vi "Read Block.vi"(8 "error in (no error)":errorcluster, 11 "Scope5761":refnum<class "Scope5782_six_channel.lvclass">) -> (0 "error out":errorcluster, 1 "#elements":i32, 2 "Data":dbl[][](array[numeric]), 3 "Scope5761":refnum<class "Scope5782_six_channel.lvclass">, 4 "FFT buffer":dbl[][](array[numeric]))   [LabVIEW 2025, in "Scope5782_six_channel.lvclass"]
uses:
  Scope5782_six_channel.lvclass
  controls/host_transfer_speed.ctl
  ScopeBase/ScopeBase.lvclass/ScopeBase.ctl
  Scope5782_six_channel.lvclass/Scope5782_six_channel.ctl
  FpgaRef/FpgaRef5761/FpgaRef5761.lvclass
  FpgaRef/FpgaRef5782/FpgaRef5782.lvclass
  ScopeBase/ScopeBase.lvclass
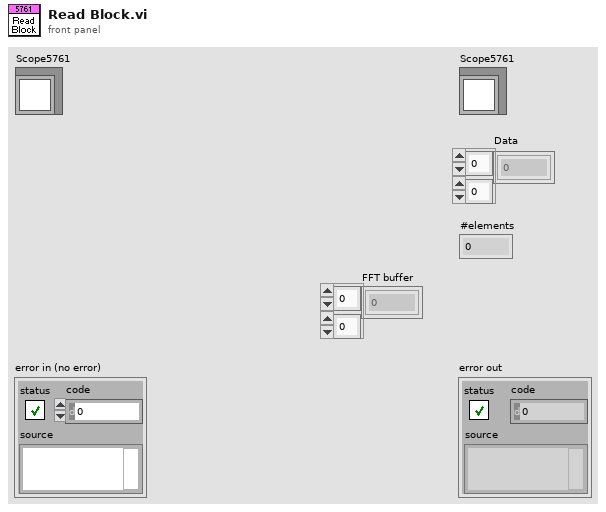
[diagram p1: front panel]
types:
  T1 = typedef "host_transfer_speed.ctl" = enum16{"Very high speed (10Ms/s)", "High speed (1Ms/s)", "Low speed (50kS/s)", "Ultra low speed (20kS/s)"}
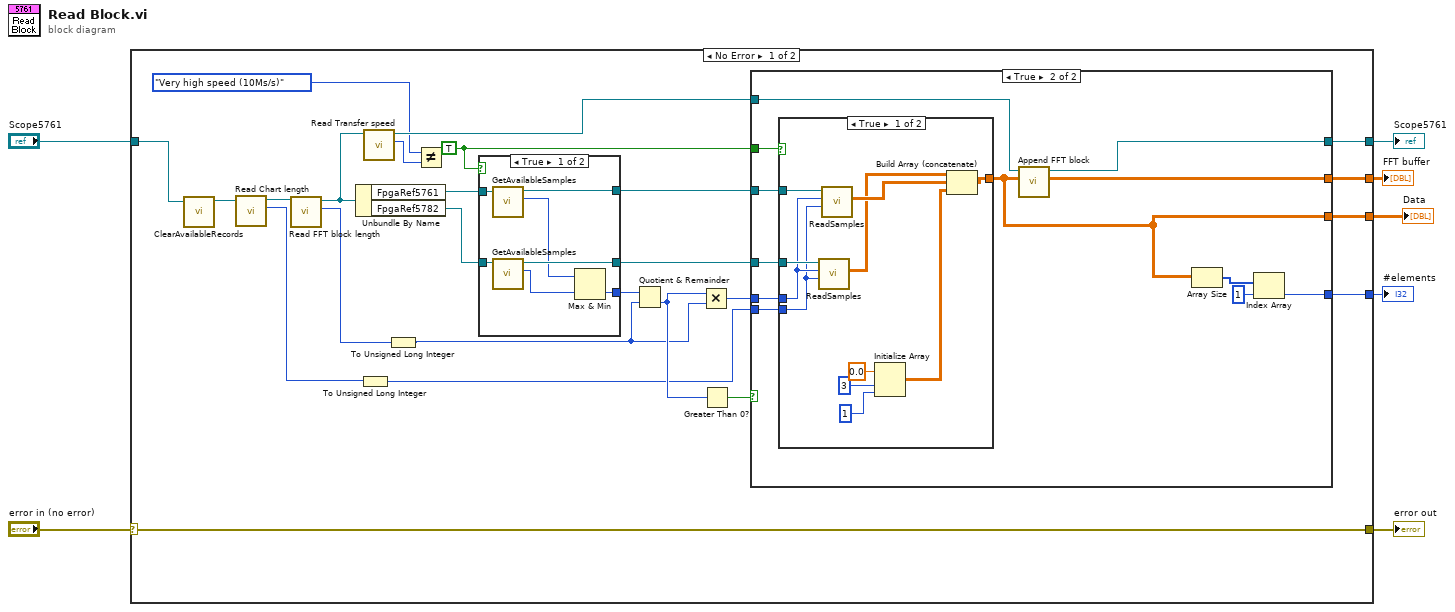
[diagram p0: block diagram]
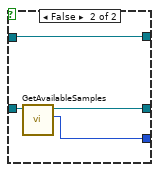
[diagram p2: hidden frame]
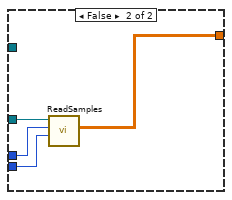
[diagram p4: hidden frame]
diagram:
  n1 = case shown="No Error" "error in (no error)" {
    selector: "error in (no error)" -> [w32 w73]
    tunnel: [w32 w73] -> w6
    tunnel: [w16 w72] -> w4
    tunnel: "Scope5761" -> [w25 w72]
    tunnel: [w31 _] -> w3
    tunnel: [w30 _] -> w2
    tunnel: [w15 _] -> w1
    frame No Error {
      w8 = TRUE
      n2 = call "ClearAvailableRecords.vi"("Scope5785_six_channel"=w25) -> ("Scope5785_six_channel out"=w23:refnum<class "Scope5782_six_channel.lvclass">)  [unwired: 9 in, 1 out]
      n3 = call "Read Chart length.vi"("ScopeBase in"=w23) -> ("Chart length"=w18:i32, "ScopeBase out"=w22:refnum<class "Scope5782_six_channel.lvclass">)  [unwired: 8 in, 1 out]
      n4 = call "Read FFT block length.vi"("ScopeBase in"=w22) -> ("FFT block length"=w14:i32, "ScopeBase out"=w12:refnum<class "Scope5782_six_channel.lvclass">)  [unwired: 8 in, 1 out]
      n5 = Unbundle By Name(w12) -> ("FpgaRef5761"=w29:refnum<class "FpgaRef5761.lvclass">, "FpgaRef5782"=w28:refnum<class "FpgaRef5782.lvclass">)
      n6 = To Unsigned Long Integer(number=w18) -> (unsigned 32bit integer=w17:u32)
      n7 = call "Read Transfer speed.vi"("ScopeBase in"=w12) -> ("Tranfer speed"=w10:T1, "ScopeBase out"=w11:refnum<class "Scope5782_six_channel.lvclass">)  [unwired: 8 in, 1 out]
      n8 = To Unsigned Long Integer(number=w14) -> (unsigned 32bit integer=w13:u32)
      n9 = Not Equal?(x=host_transfer_speed."Very high speed (10Ms/s)" ("y"), y=w10) -> ()  [unwired: 1 out]
      n10 = case shown="True" w8 {
        tunnel: w29 -> [w39 w41]
        tunnel: w28 -> [w38 w43]
        tunnel: [w36 w41] -> w27
        tunnel: [w35 w42] -> w26
        tunnel: [w33 w40] -> w24
        frame True {
          n11 = call-dynamic "GetAvailableSamples.vi"("FpgaRef5761 In"=w39) -> ("available"=w34:u32, "FpgaRef5761 Out"=w36:refnum<class "FpgaRef5761.lvclass">)  [unwired: 8 in, 1 out]
          n12 = call-dynamic "GetAvailableSamples.vi"("FpgaRef5782 in"=w38) -> ("available"=w37:u32, "FpgaRef5782 out"=w35:refnum<class "FpgaRef5782.lvclass">)  [unwired: 8 in, 1 out]
          n13 = Max & Min(x=w34, y=w37) -> (min(x,y)=w33:u32)  [unwired: 1 out]
        }
        frame False {
          n14 = call-dynamic "GetAvailableSamples.vi"("FpgaRef5782 in"=w43) -> ("available"=w40:u32, "FpgaRef5782 out"=w42:refnum<class "FpgaRef5782.lvclass">)  [unwired: 8 in, 1 out]
        }
      }
      n15 = Quotient & Remainder(x=w24, y=w13) -> (floor(x/y)=w20:u32)  [unwired: 1 out]
      n16 = Multiply(x=w20, y=w13) -> (x*y=w19:u32)
      n17 = Greater Than 0?(x=w20) -> (x > 0?=w21:bool)
      n18 = case shown="True" w21 {
        tunnel: [_ w47] -> w31
        tunnel: [_ w54] -> w30
        tunnel: w19 -> [_ w51]
        tunnel: w17 -> [_ w50]
        tunnel: w27 -> [_ w53]
        tunnel: w26 -> [_ w52]
        tunnel: w11 -> [w44 w49]
        tunnel: [w44 w48] -> w16
        tunnel: [_ w46] -> w15
        tunnel: w8 -> [_ w45]
        frame False {
        }
        frame True {
          n19 = case shown="True" w45 {
            tunnel: w53 -> [w67 _]
            tunnel: w52 -> [w66 w71]
            tunnel: w51 -> [w65 w70]
            tunnel: w50 -> [w62 w69]
            tunnel: [w61 w68] -> w47
            frame True {
              n20 = call-dynamic "ReadSamples.vi"("Max num samples to keep"=w62, "Num samples to read"=w65, "FpgaRef5782 in"=w66) -> ("Data"=w63:dbl[][])  [unwired: 6 in, 2 out]
              n21 = call-dynamic "ReadSamples.vi"("Max num samples to keep"=w62, "Num samples to read"=w65, "FpgaRef5761 In"=w67) -> ("Data"=w64:dbl[][])  [unwired: 6 in, 2 out]
              n22 = Initialize Array(0.0 ("element"), 3 ("dimension size"), 1 ("dimension size")) -> (w57:dbl[][])
              n23 = Build Array (concatenate)(w63, w64, w57) -> (w61:dbl[][])
            }
            frame False {
              n24 = call-dynamic "ReadSamples.vi"("Max num samples to keep"=w69, "Num samples to read"=w70, "FpgaRef5782 in"=w71) -> ("Data"=w68:dbl[][])  [unwired: 6 in, 2 out]
            }
          }
          n25 = call "Append FFT block.vi"("new data"=w47, "ScopeBase in"=w49) -> ("FFT buffer"=w46:dbl[][], "ScopeBase out"=w48:refnum<class "Scope5782_six_channel.lvclass">)  [unwired: 7 in, 1 out]
          n26 = Array Size(array=w47) -> (size(s)=w56:i32[])
          n27 = Index Array(array=w56, index=1) -> (element=w54:i32)
        }
      }
    }
    frame Error {
    }
  }
  "error out" <- w6
  "Scope5761" <- w4
  "Data" <- w3
  "#elements" <- w2
  "FFT buffer" <- w1
